vi "getEdges.vi"(0 "reference":refnum<class "Graph.lvclass">, 5 "error in (no error)":errorcluster) -> (14 "reference out":refnum<class "Graph.lvclass">, 15 "edges":refnum<class "AbstractEdge.lvclass">[](array[class]), 19 "error out":errorcluster)   [LabVIEW 2012, in "Graph.lvclass"]
doc: "public Collection getEdges()"
uses:
  <resource>/Framework/Providers/Open_GDS/UML/Graph_class/Graph.lvclass
  <resource>/Framework/Providers/Open_GDS/UML/AbstractEdge_class/AbstractEdge.lvclass
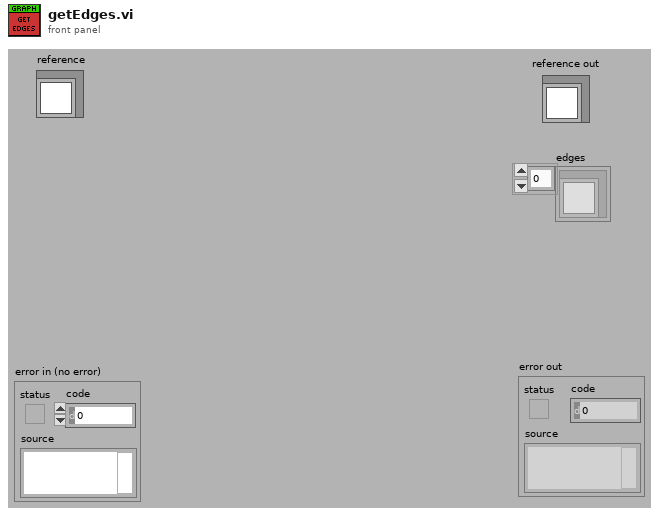
[diagram p1: front panel]
types:
  T1 = typedef "Graph.lvclass/ObjectAttributes.ctl" = cluster{"nodes":refnum<class "AbstractNode.lvclass">[], "edges":refnum<class "AbstractEdge.lvclass">[], "nodesToBeRemoved":refnum<class "AbstractNode.lvclass">[], "edgesToBeRemoved":refnum<class "AbstractEdge.lvclass">[], "needsLayout":bool, "LayoutNodes":refnum<class "AbstractNode.lvclass">[]}
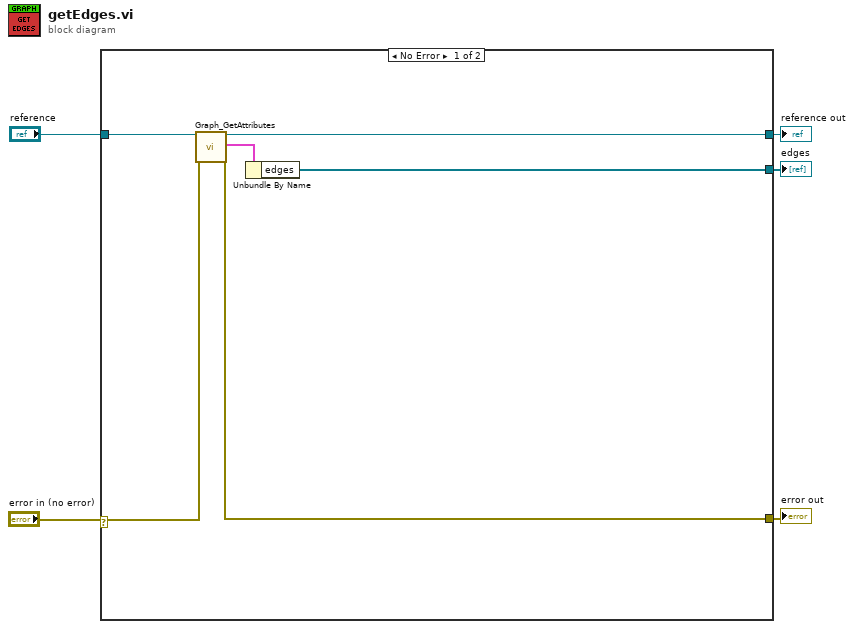
[diagram p0: block diagram]
diagram:
  n1 = case shown="No Error" "error in (no error)" {
    selector: "error in (no error)" -> [w8 w12]
    tunnel: "reference" -> [w11 w13]
    tunnel: [w10 w12] -> w4
    tunnel: [w9 w13] -> w3
    tunnel: [w7 _] -> w1
    frame No Error {
      n2 = call <resource>:"Graph_GetAttributes.vi"("reference in"=w11, "error in (no error)"=w8) -> ("reference out"=w9:refnum<class "Graph.lvclass">, "Attributes"=w6:T1, "error out"=w10:errorcluster)  [unwired: 15 out]
      n3 = Unbundle By Name(w6) -> ("edges"=w7:refnum<class "AbstractEdge.lvclass">[])
    }
    frame Error {
    }
  }
  "reference out" <- w3
  "error out" <- w4
  "edges" <- w1
